vi "update config.vi"(8 "error in (no error)":errorcluster, 10 "user configurations":T2={"vst_device"=["VST_1", "VST_2"], "RF gain "=10.0, "buffer size"=524288, "center frequency (Hz) "=1000000000.0, "P2P sample rate"=200000000.0, "mode"=enum."5785 - 2*180MHz", "devicess"=["IF_transiver_0", "IF_transiver_1", "IF_transiver_2"], "file paths"=[path "C:/Users/PXIe8108_Demo/Documents/CHAIM DATA/chaim/5785_sync_for_elbit/data/pdw_test_file.tdms", path "C:/Users/PXIe8108_Demo/Documents/CHAIM DATA/chaim/5785_sync_for_elbit/data/pdw_test_file_1.tdms", path "C:/Users/PXIe8108_Demo/Documents/CHAIM DATA/chaim/5785_sync_for_elbit/data/pdw_test_file_2.tdms", path "C:/Users/PXIe8108_Demo/Documents/CHAIM DATA/chaim/5785_sync_for_elbit/data/pdw_test_file_3.tdms", path "C:/Users/PXIe8108_Demo/Documents/CHAIM DATA/chaim/5785_sync_for_elbit/data/pdw_test_file_4.tdms"], "gen for df"=FALSE}, 11 "p2p vst in":refnum<class "p2p vst.lvclass">) -> (0 "error out":errorcluster, 1 "min frequency":dbl, 2 "max frequency":dbl, 3 "p2p vst out":refnum<class "p2p vst.lvclass">)   [LabVIEW 2021, in "p2p vst.lvclass"]
uses:
  p2p vst.lvclass
  <vilib>/userdefined/High Color/nirio_resource_hc.ctl
  p2p vst.lvclass/p2p vst.ctl
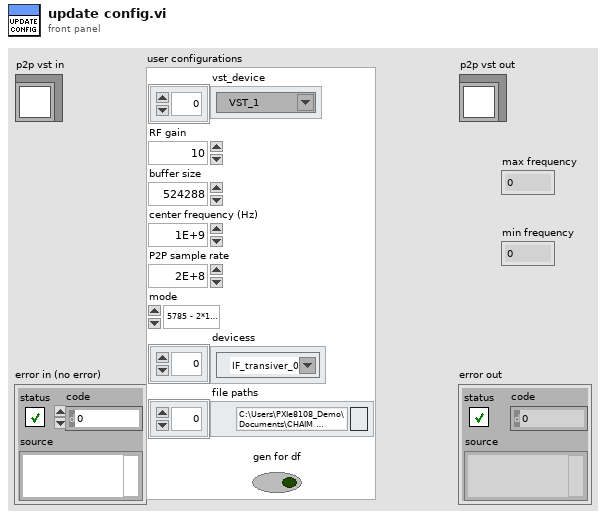
[diagram p1: front panel]
types:
  T1 = typedef "nirio_resource_hc.ctl" = tag
  T2 = cluster{"vst_device":refnum<k15>[], "RF gain ":dbl, "buffer size":u32, "center frequency (Hz) ":dbl, "P2P sample rate":dbl, "mode":enum16{"USRP - 180MHz", "5785 - 2*180MHz", "5785 - 3.2GHz", "P2P - VST"}, "devicess":T1[], "file paths":path[], "gen for df":bool}
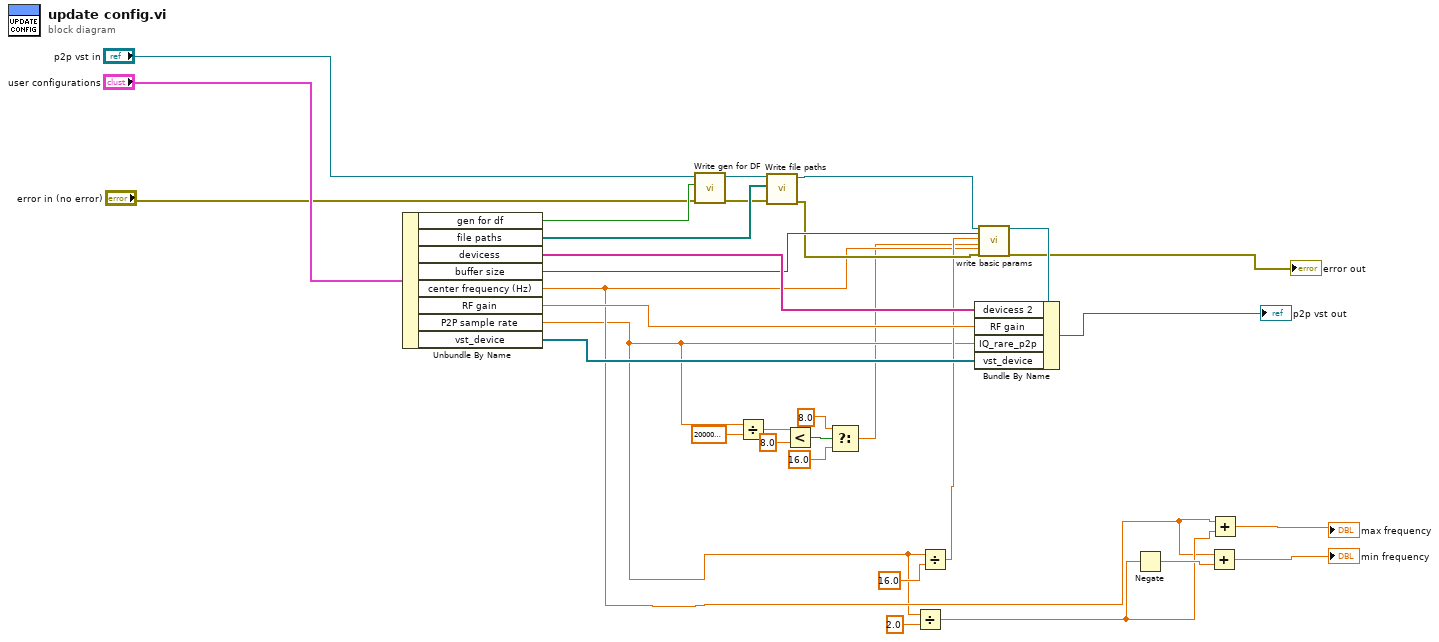
[diagram p0: block diagram]
diagram:
  n1 = Unbundle By Name("user configurations") -> ("gen for df"=w26:bool, "file paths"=w29:path[], "devicess"=w32:T1[], "buffer size"=w31:u32, "center frequency (Hz)"=w9:dbl, "RF gain"=w23:dbl, "P2P sample rate"=w8:dbl, "vst_device"=w17:refnum<k15>[])
  n2 = call-dynamic "Write gen for DF.vi"("error in (no error)"="error in (no error)", "gen for DF"=w26, "device_type in"="p2p vst in") -> ("error out"=w25:errorcluster, "device_type out"=w27:refnum<class "p2p vst.lvclass">)  [unwired: 7 in]
  n3 = Divide(x=w8, y=200000000.0) -> (x/y=w6:dbl)
  n4 = call-dynamic "Write file paths.vi"("error in (no error)"=w25, "file paths"=w29, "device_type in"=w27) -> ("error out"=w24:errorcluster, "device_type out"=w28:refnum<class "p2p vst.lvclass">)  [unwired: 7 in]
  n5 = Less?(x=w6, y=8.0) -> (x < y?=w4:bool)
  n6 = Select(t=8.0, s=w4, f=16.0 ("Fs  FPGA")) -> (s? t:f=w3:dbl)
  n7 = Divide(x=w8, y=2.0) -> (x/y=w15:dbl)
  n8 = Divide(x=w8, y=16.0 ("Fs  FPGA")) -> (x/y=w10:dbl)
  n9 = call-dynamic "write basic params.vi"("device_type in"=w28, "buffer size"=w31, "Fs  FPGA"=w10, "SPC"=w3, "center frequency (Hz)"=w9, "error in (no error)"=w24) -> ("device_type out"=w30:refnum<class "p2p vst.lvclass">, "error out"=→"error out":errorcluster)  [unwired: 12 in]
  n10 = Bundle By Name(cluster=w30, "devicess 2"=w32, "RF gain"=w23, "IQ_rare_p2p"=w8, "vst_device"=w17) -> (→"p2p vst out":refnum<class "p2p vst.lvclass">)
  n11 = Negate(x=w15) -> (-x=w16:dbl)
  n12 = Add(x=w9, y=w16) -> (x+y=→"min frequency":dbl)
  n13 = Add(x=w9, y=w15) -> (x+y=→"max frequency":dbl)
